vi "MixAndDownsample.vi"(9 "Sine in":fxp<+/-,16,0>[](array[numeric])=[0.0, 0.0, 0.0, 0.0], 10 "Cosine in":fxp<+/-,16,0>[](array[numeric])=[0.0, 0.0, 0.0, 0.0], 11 "Signal Input":i16[](array[numeric])=[0, 0, 0, 0]) -> (0 "data valid":bool, 1 "Q out":fxp<+/-,20,16>, 2 "I out":fxp<+/-,20,16>)   [LabVIEW 2013]
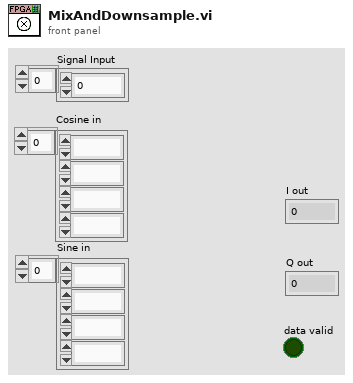
[diagram p1: front panel]
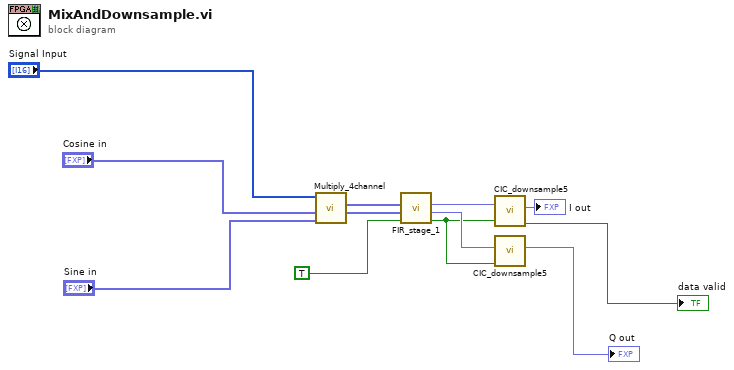
[diagram p0: block diagram]
diagram:
  n1 = call "Multiply_4channel.vi"("DDS Sine"="Sine in", "DDS Cosine"="Cosine in", "Signal Input"="Signal Input") -> ("Q output"=w8:fxp<+/-,16,14>[], "I output"=w9:fxp<+/-,16,14>[])  [unwired: 7 in]
  n2 = call "FIR_stage_1.vi"("data valid in"=TRUE ("valid in"), "Q in"=w8, "I in"=w9) -> ("data valid out"=w1:bool, "Q out"=w6:fxp<+/-,20,16>, "I out"=w7:fxp<+/-,20,16>)  [unwired: 6 in]
  n3 = call "CIC_downsample5.vi"("valid in"=w1, "din"=w7) -> ("valid out"=→"data valid":bool, "dout"=→"I out":fxp<+/-,20,16>)  [unwired: 8 in]
  n4 = call "CIC_downsample5.vi"("valid in"=w1, "din"=w6) -> ("dout"=→"Q out":fxp<+/-,20,16>)  [unwired: 8 in, 1 out]
